vi "Run.vi"(8 "error in (no error)":errorcluster, 11 "Telemetry in":refnum<class "Telemetry.lvclass">) -> (0 "error out":errorcluster, 3 "Telemetry out":refnum<class "Telemetry.lvclass">)   [LabVIEW 2018, in "Telemetry.lvclass"]
uses:
  Telemetry.lvclass
  Telemetry.lvclass/Telemetry.ctl
  Device/Device.lvclass
  StateMachine/State Machine.lvclass
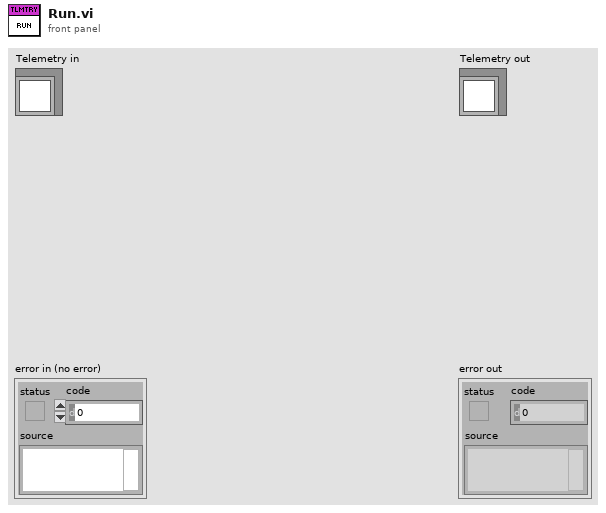
[diagram p1: front panel]
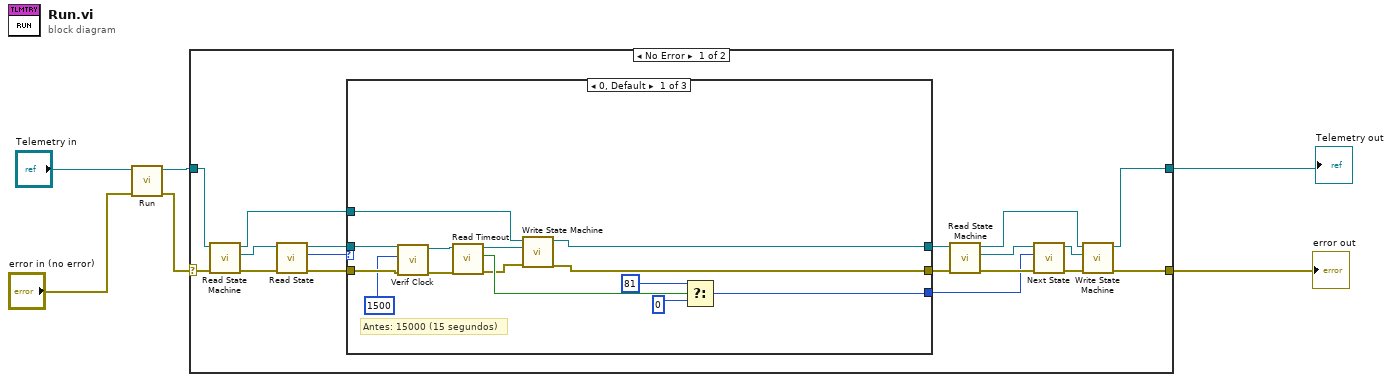
[diagram p0: block diagram]
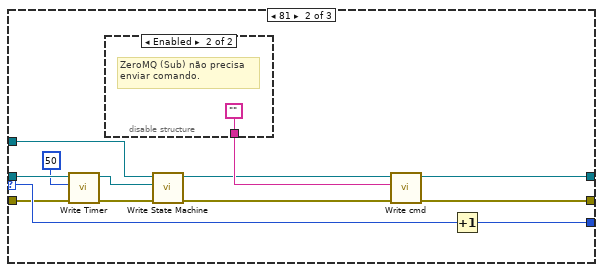
[diagram p2: hidden frame]
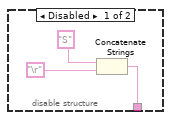
[diagram p3: hidden frame]
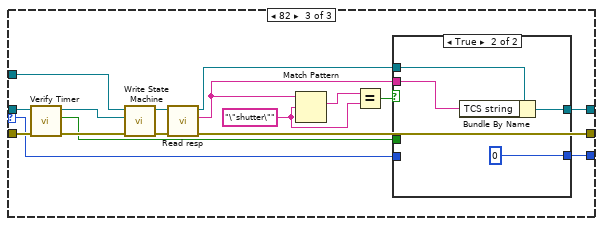
[diagram p4: hidden frame]
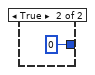
[diagram p6: hidden frame]
diagram:
  n1 = call-parent "Run.vi"("error in (no error)"="error in (no error)", "Device in"="Telemetry in") -> ("error out"=w3:errorcluster, "Device out"=w4:refnum<class "Telemetry.lvclass">)  [unwired: 8 in]
  n2 = case shown="No Error" w3 {
    selector: w3 -> [w23 w84]
    tunnel: [w15 w84] -> w1
    tunnel: w4 -> [w24 w83]
    tunnel: [w14 w83] -> w2
    frame No Error {
      n3 = call-dynamic "Read State Machine.vi"("error in (no error)"=w23, "Device in"=w24) -> ("error out"=w21:errorcluster, "State Machine.lvclass"=w22:refnum<class "State Machine.lvclass">, "Device out"=w12:refnum<class "Telemetry.lvclass">)  [unwired: 7 in]
      n4 = call-dynamic "Read State.vi"("error in (no error)"=w21, "State Machine in"=w22) -> ("error out"=w11:errorcluster, "State"=w13:i32, "State Machine out"=w7:refnum<class "State Machine.lvclass">)  [unwired: 7 in]
      n5 = case shown="0, Default" w13 {
        selector: w13 -> [_ w51 w61]
        tunnel: w12 -> [w30 w46 w66]
        tunnel: w11 -> [w33 w44 w64]
        tunnel: [w26 w39 w70] -> w10
        tunnel: [w27 w40 w71] -> w9
        tunnel: [w38 w50 w69] -> w8
        tunnel: w7 -> [w32 w48 w68]
        frame 0, Default {
          # "Antes: 15000 (15 segundos)"
          n6 = call-dynamic "Verif Clock.vi"("error in (no error)"=w33, "period (ms)"=u32 1500 ("period"), "State Machine in"=w32) -> ("error out"=w34:errorcluster, "State Machine out"=w31:refnum<class "State Machine.lvclass">)  [unwired: 6 in, 1 out]
          n7 = call-dynamic "Read Timeout.vi"("error in (no error)"=w34, "State Machine in"=w31) -> ("error out"=w28:errorcluster, "Timeout"=w35:bool, "State Machine out"=w29:refnum<class "State Machine.lvclass">)  [unwired: 7 in]
          n8 = call-dynamic "Write State Machine.vi"("error in (no error)"=w28, "State Machine.lvclass"=w29, "Device in"=w30) -> ("error out"=w26:errorcluster, "Device out"=w27:refnum<class "Telemetry.lvclass">)  [unwired: 7 in]
          n9 = Select(t=81 ("State"), s=w35, f=0 ("State")) -> (s? t:f=w38:i32)
        }
        frame 81 {
          n10 = call-dynamic "Write Timer.vi"("error in (no error)"=w44, "Timer"=u32 50, "State Machine in"=w48) -> ("error out"=w43:errorcluster, "State Machine out"=w42:refnum<class "State Machine.lvclass">)  [unwired: 7 in]
          n11 = disable-structure shown="Enabled" {
            disable-tunnel: [w52 "" ("cmd")] -> w49
            frame Disabled {
              n12 = Concatenate Strings("S" ("cmd"), "\r") -> (w52:string)
            }
            frame Enabled {
              # "ZeroMQ (Sub) não precisa\nenviar comando."
            }
          }
          n13 = call-dynamic "Write State Machine.vi"("error in (no error)"=w43, "State Machine.lvclass"=w42, "Device in"=w46) -> ("error out"=w41:errorcluster, "Device out"=w45:refnum<class "Telemetry.lvclass">)  [unwired: 7 in]
          n14 = call-dynamic "Write cmd.vi"("error in (no error)"=w41, "cmd"=w49, "Device in"=w45) -> ("error out"=w39:errorcluster, "Device out"=w40:refnum<class "Telemetry.lvclass">)  [unwired: 7 in]
          n15 = Increment(x=w51) -> (x+1=w50:i32)
        }
        frame 82 {
          w58 = "\"shutter\"" ("regular expression")
          n16 = call "Verify Timer.vi"("error in (no error)"=w64, "State Machine in"=w68) -> ("error out"=w65:errorcluster, "timeout"=w56:bool, "State Machine out"=w67:refnum<class "State Machine.lvclass">)  [unwired: 7 in]
          n17 = call-dynamic "Write State Machine.vi"("error in (no error)"=w65, "State Machine.lvclass"=w67, "Device in"=w66) -> ("error out"=w62:errorcluster, "Device out"=w63:refnum<class "Telemetry.lvclass">)  [unwired: 7 in]
          n18 = call-dynamic "Read resp.vi"("error in (no error)"=w62, "Device in"=w63) -> ("error out"=w70:errorcluster, "resp"=w57:string, "Device out"=w72:refnum<class "Telemetry.lvclass">)  [unwired: 7 in]
          n19 = Match Pattern(string=w57, regular expression=w58) -> (match substring=w59:string)  [unwired: 1 in, 3 out]
          n20 = Equal?(x=w59, y=w58) -> (x = y?=w60:bool)
          n21 = case shown="True" w60 {
            tunnel: w72 -> [w76 w82]
            tunnel: [w76 w81] -> w71
            tunnel: [w74 0] -> w69
            tunnel: w61 -> [w75 _]
            tunnel: w57 -> [_ w79]
            tunnel: w56 -> [w73 _]
            frame False {
              n22 = case shown="False" w73 {
                tunnel: w75 -> [w77 _]
                tunnel: [w77 0 ("State")] -> w74
                frame False {
                }
                frame True {
                }
              }
            }
            frame True {
              n23 = Bundle By Name(cluster=w82, "TCS string"=w79) -> (w81:refnum<class "Telemetry.lvclass">)
            }
          }
        }
      }
      n24 = call-dynamic "Read State Machine.vi"("error in (no error)"=w10, "Device in"=w9) -> ("error out"=w17:errorcluster, "State Machine.lvclass"=w19:refnum<class "State Machine.lvclass">, "Device out"=w18:refnum<class "Telemetry.lvclass">)  [unwired: 7 in]
      n25 = call "Next State.vi"("error in (no error)"=w17, "New_State"=w8, "State Machine in"=w19) -> ("error out"=w16:errorcluster, "State Machine out"=w20:refnum<class "State Machine.lvclass">)  [unwired: 7 in]
      n26 = call-dynamic "Write State Machine.vi"("error in (no error)"=w16, "State Machine.lvclass"=w20, "Device in"=w18) -> ("error out"=w15:errorcluster, "Device out"=w14:refnum<class "Telemetry.lvclass">)  [unwired: 7 in]
    }
    frame Error {
    }
  }
  "error out" <- w1
  "Telemetry out" <- w2
